vi "Module - Setting Page.vi"() -> ()   [LabVIEW 2020]
uses:
  Control/State - Setting.ctl
  Control/State - eFGV.ctl
  Control/Button Strip.ctl
  Control/Config File Selection.ctl
panel:
  out "error out":errorcluster
  in  "error in (no error)":errorcluster
  out "Site Name":string="SETTING"
  in  "MYSQL DATABASE":T1
  in  "MODBUS TCP IP":T2
  in  "setting_save_mysql":bool
  in  "setting_save":bool
  # "DB_CONNECTION :"
  # "DB_HOST :"
  # "DB_PORT  :"
  # "DB_DATABASE  :"
  # "DB_USERNAME  :"
  # "DB_PASSWORD  :"
  # "INTERVAL  :"
  # "SB-01"
  # "IP ADDRESS"
  # "PORT"
  # "SB-02"
  # "IP ADDRESS"
  # "PORT"
  # "SI-M"
  # "IP ADDRESS"
  # "PORT"
  # "SI-01"
  # "IP ADDRESS"
  # "PORT"
  # "DATA MANAGER"
  # "IP ADDRESS"
  # "PORT"
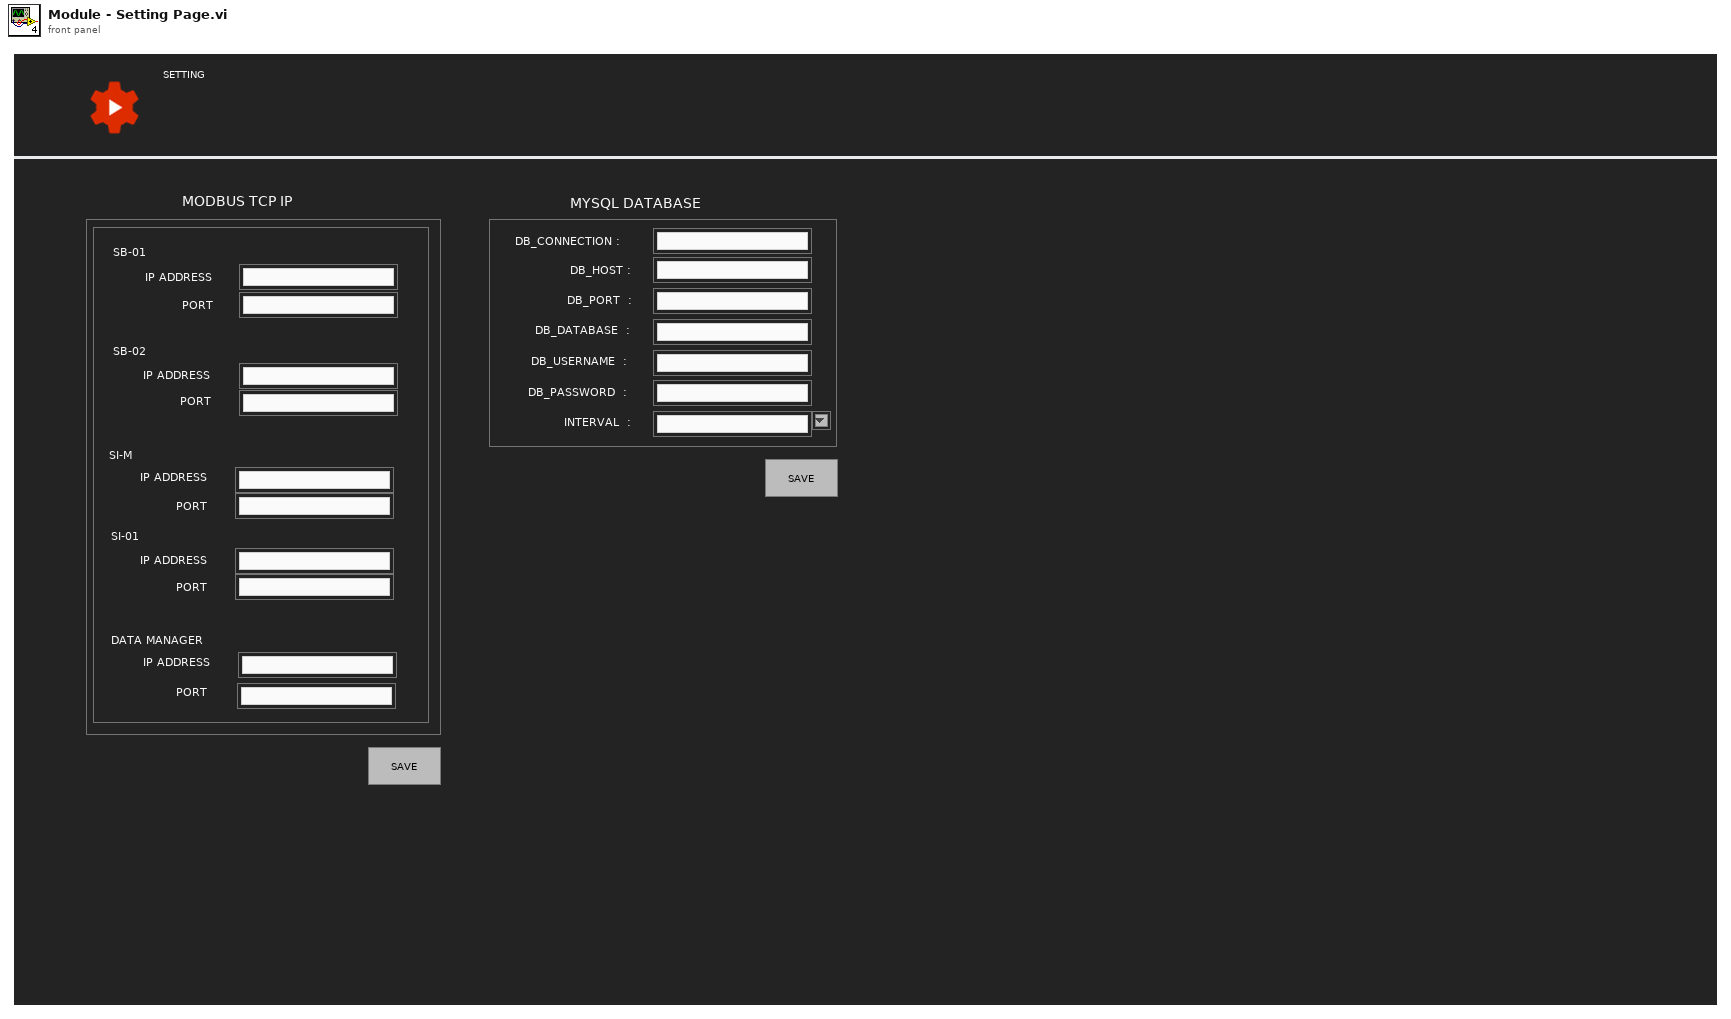
[diagram p1: front panel]
types:
  T1 = cluster{"db_connection":string, "db_host":string, "db_port":string, "db_database":string, "db_username":string, "db_pwd":string, "Interval":string}
  T2 = cluster{"DM-PORT":string, "DM-IPADDRESS":string, "SB-01-IPADDRESS":string, "SB-01-PORT":string, "SB-02-IPADDRESS":string, "SB-02-PORT":string, "SI-M-IPADDRESS":string, "SI-M-PORT":string, "SI-01-IPADDRESS":string, "SI-01-PORT":string}
  T3 = cluster{"Timeout":i32, "Modbus Config":string[][], "SQL Config":string[][]}
  T4 = typedef "State - Setting.ctl" = enum16{"Init module", "Register event", "Idle", "Read Config File", "Repopulate Indicator", "Save Modbus Settings", "Save SQL Settings", "Unregister event", "Close module"}
  T5 = typedef "Button Strip.ctl" = enum32{"Home", "Setting", "Alert", "Save", "Chart"}
  T6 = typedef "Config File Selection.ctl" = enum16{"Modbus", "SQL", "General"}
  T7 = typedef "State - eFGV.ctl" = enum16{"Init", "Read", "Write", "Close"}
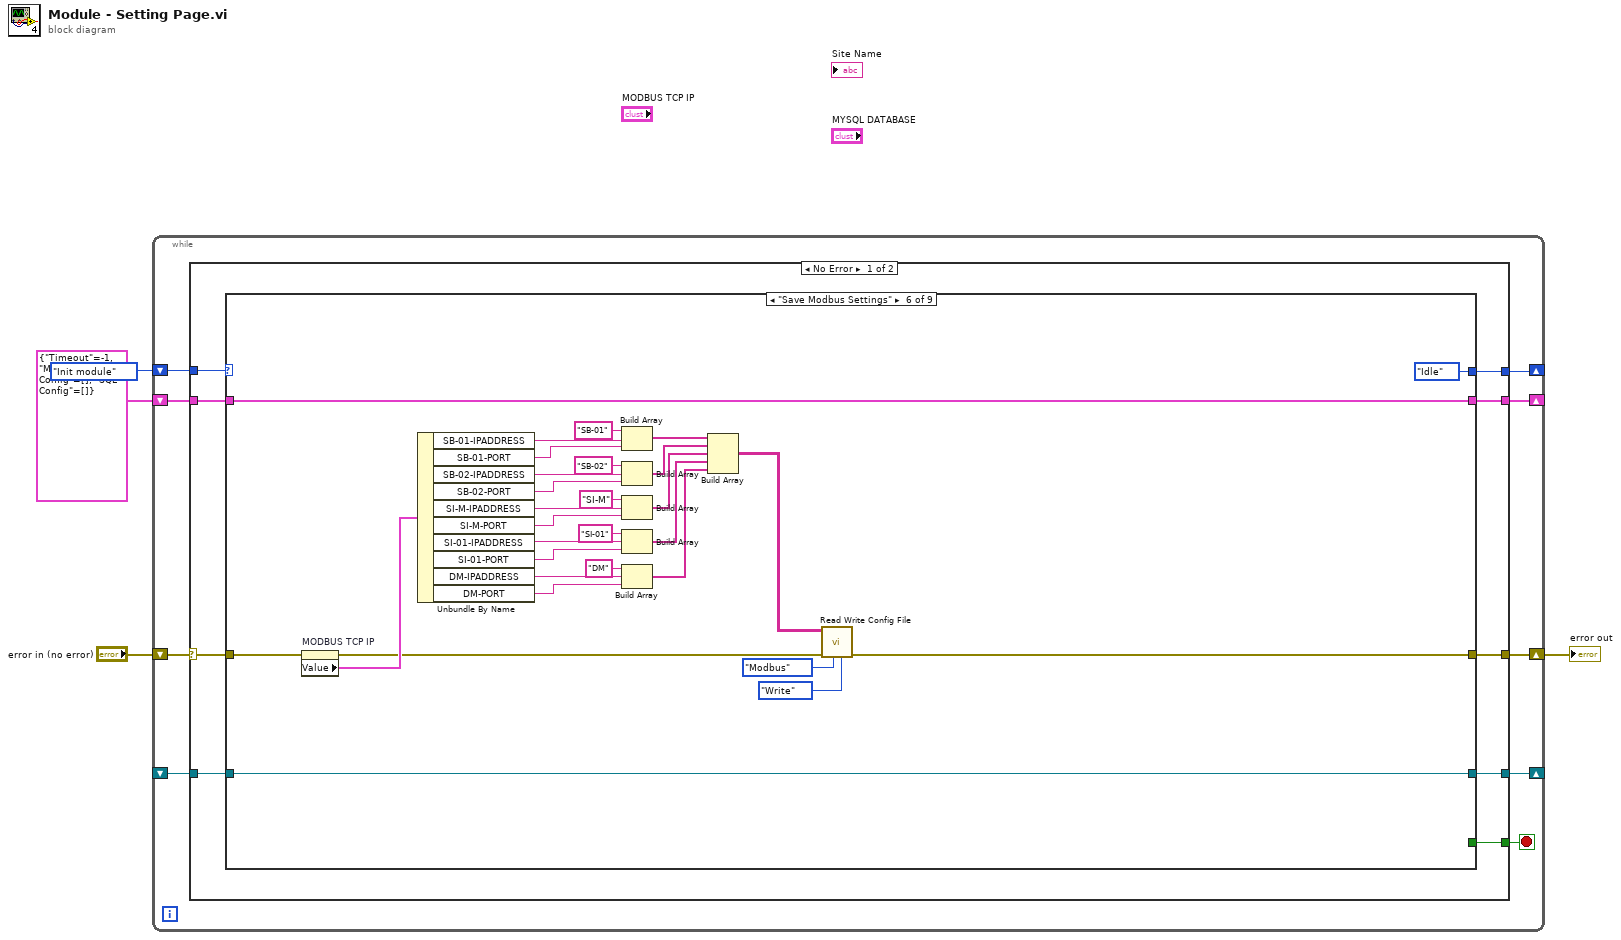
[diagram p0: block diagram]
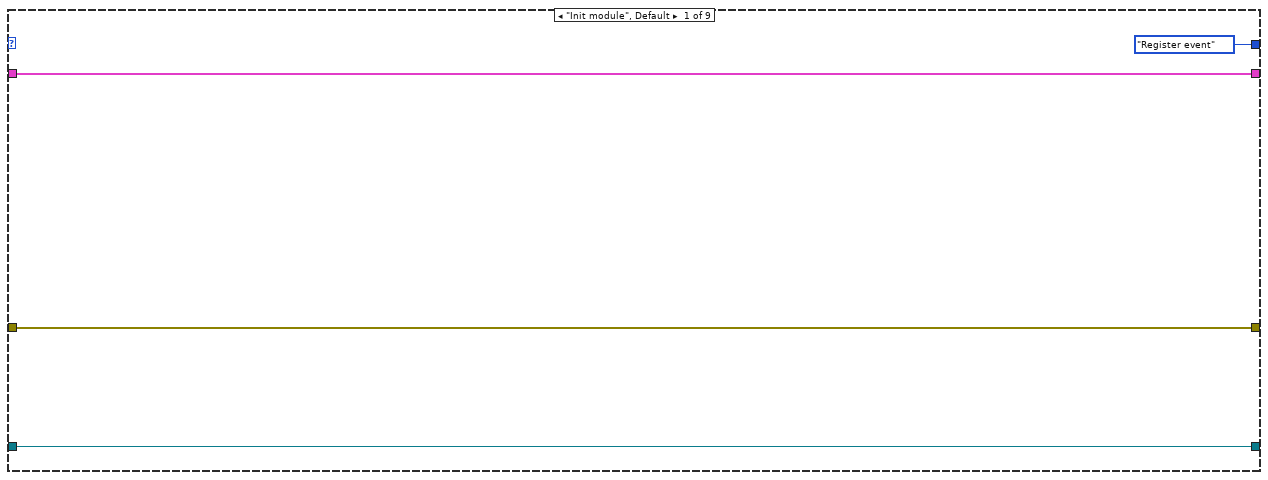
[diagram p2: hidden frame]
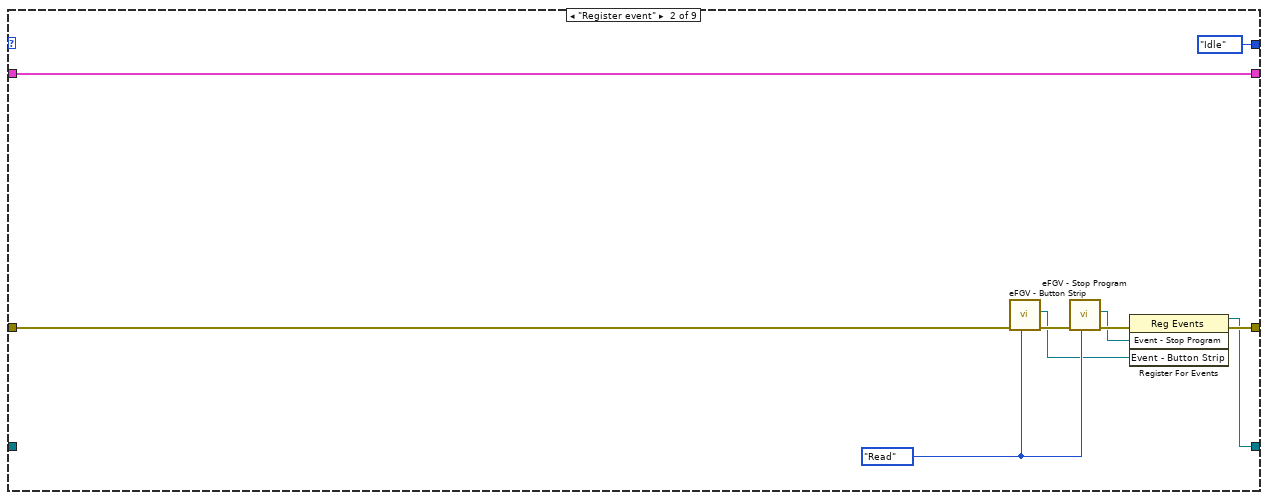
[diagram p3: hidden frame]
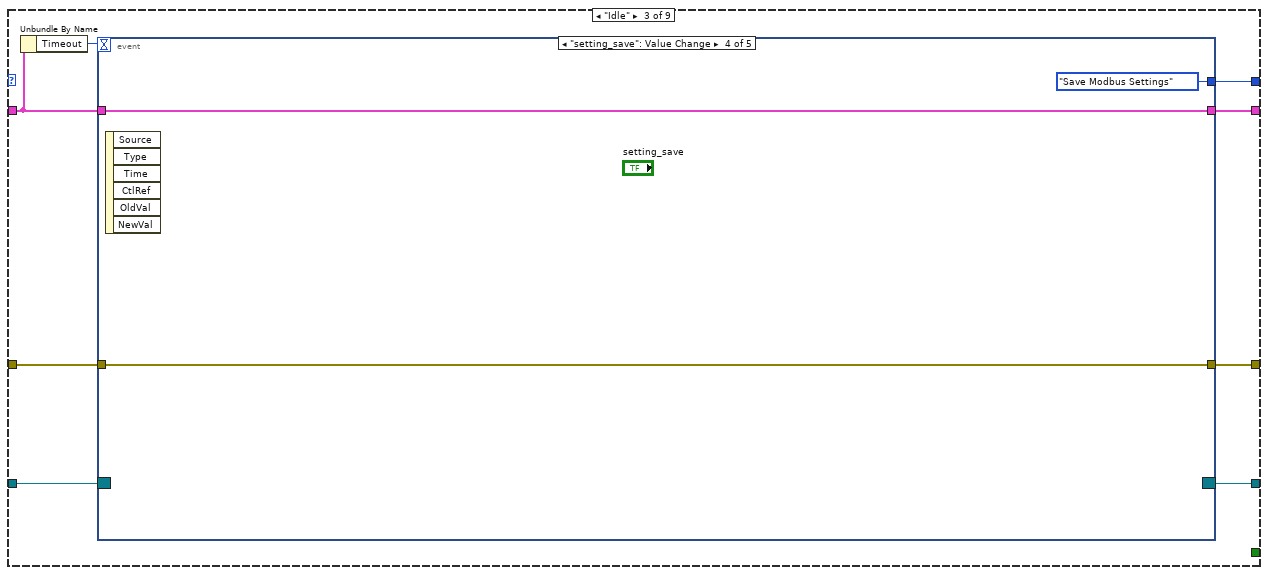
[diagram p4: hidden frame]
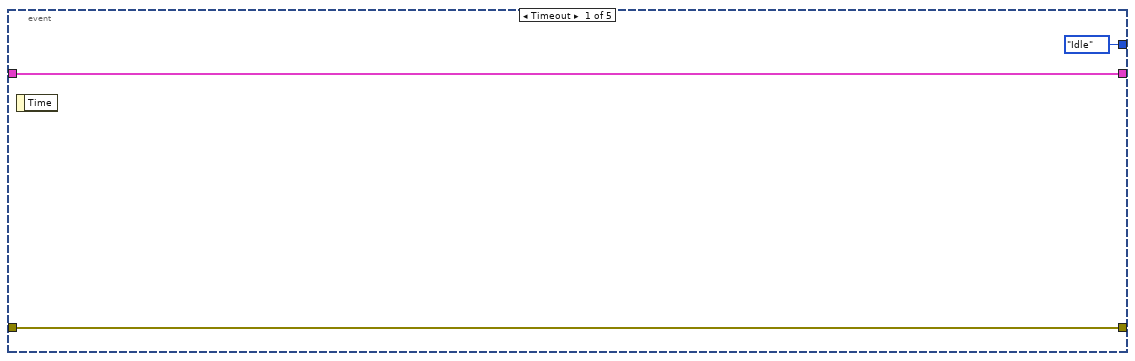
[diagram p5: hidden frame]
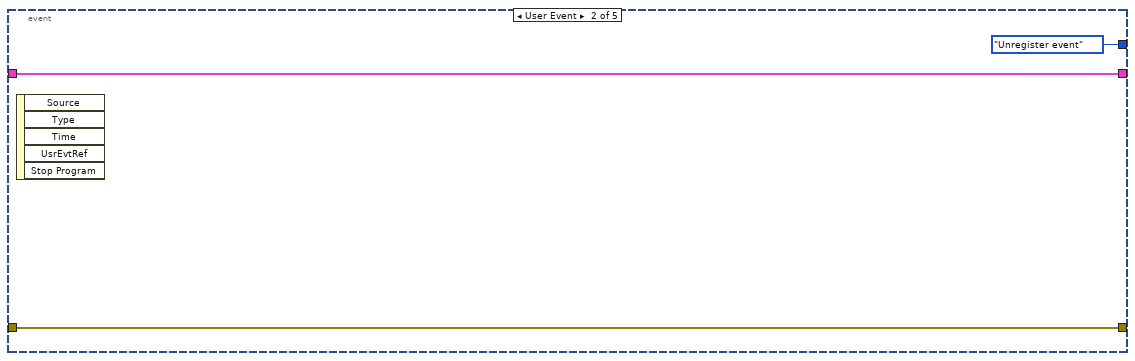
[diagram p6: hidden frame]
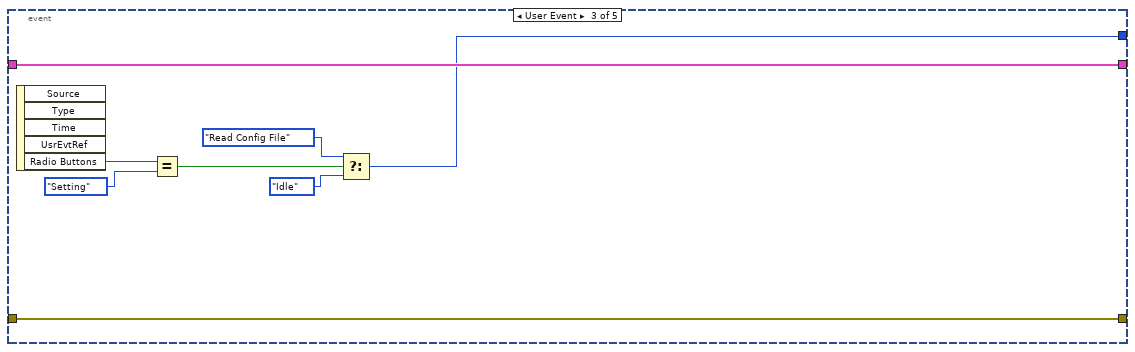
[diagram p7: hidden frame]
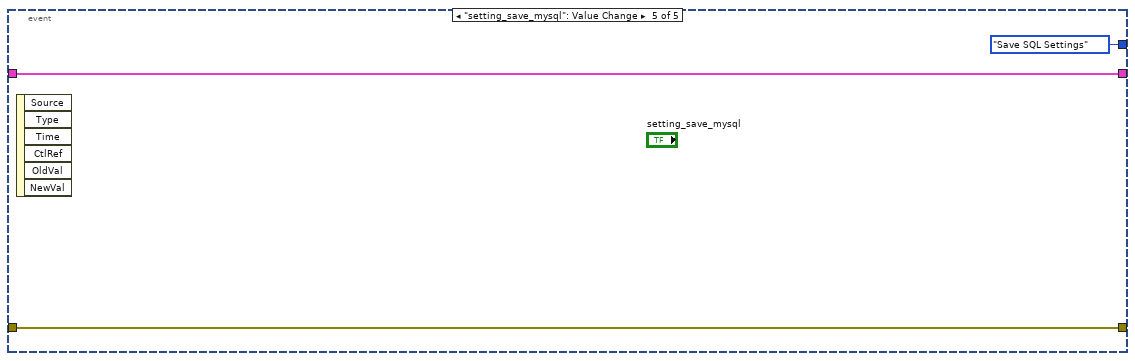
[diagram p8: hidden frame]
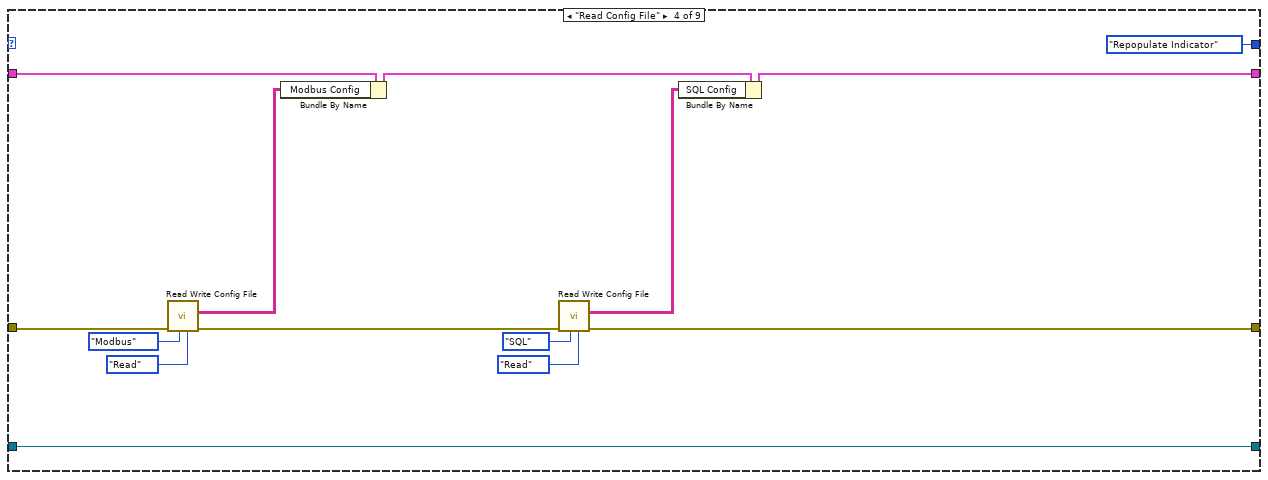
[diagram p9: hidden frame]
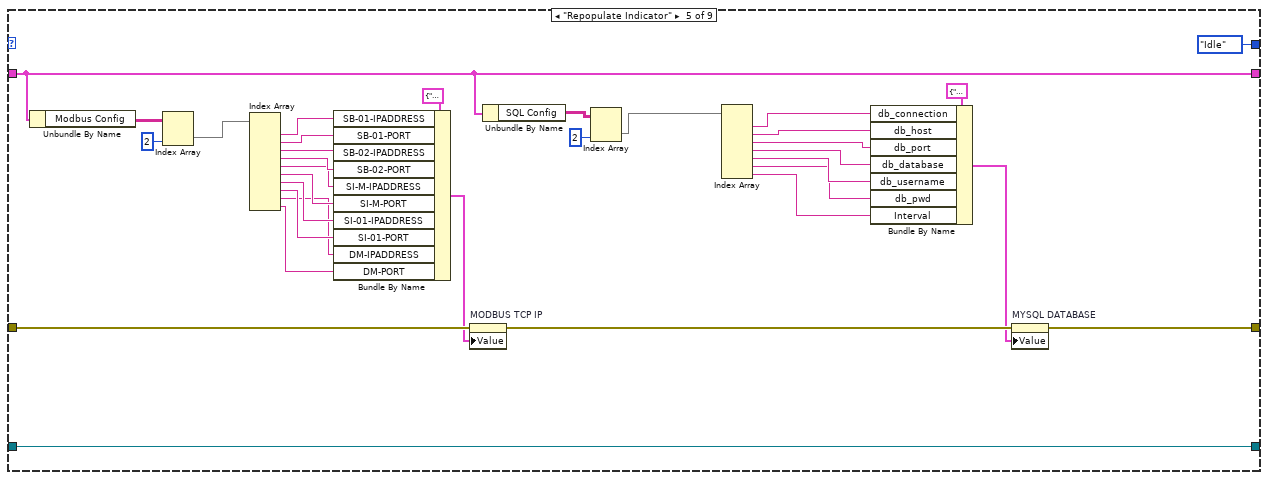
[diagram p10: hidden frame]
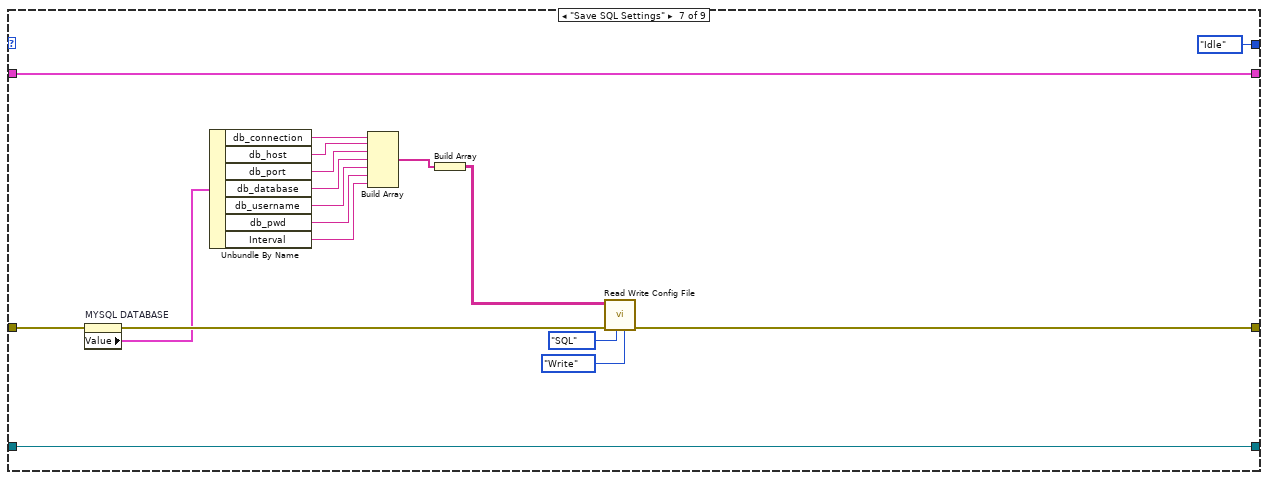
[diagram p11: hidden frame]
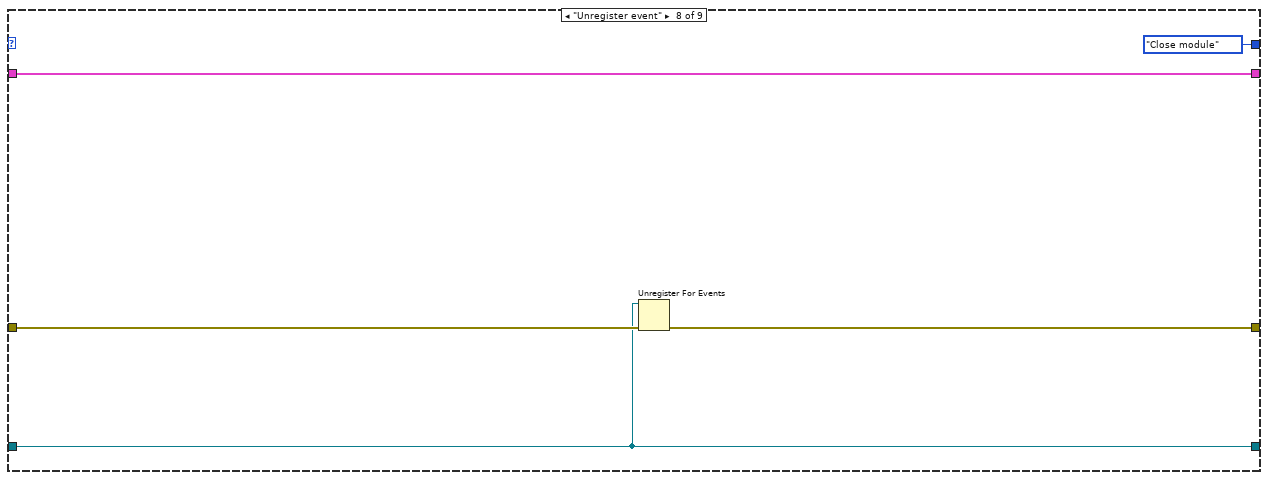
[diagram p12: hidden frame]
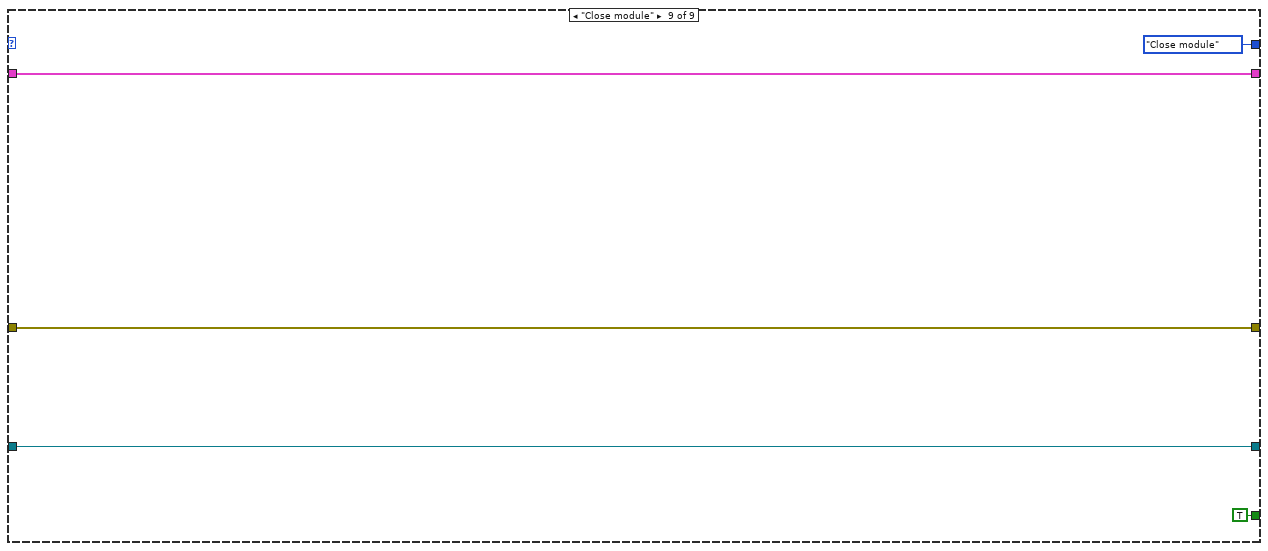
[diagram p13: hidden frame]
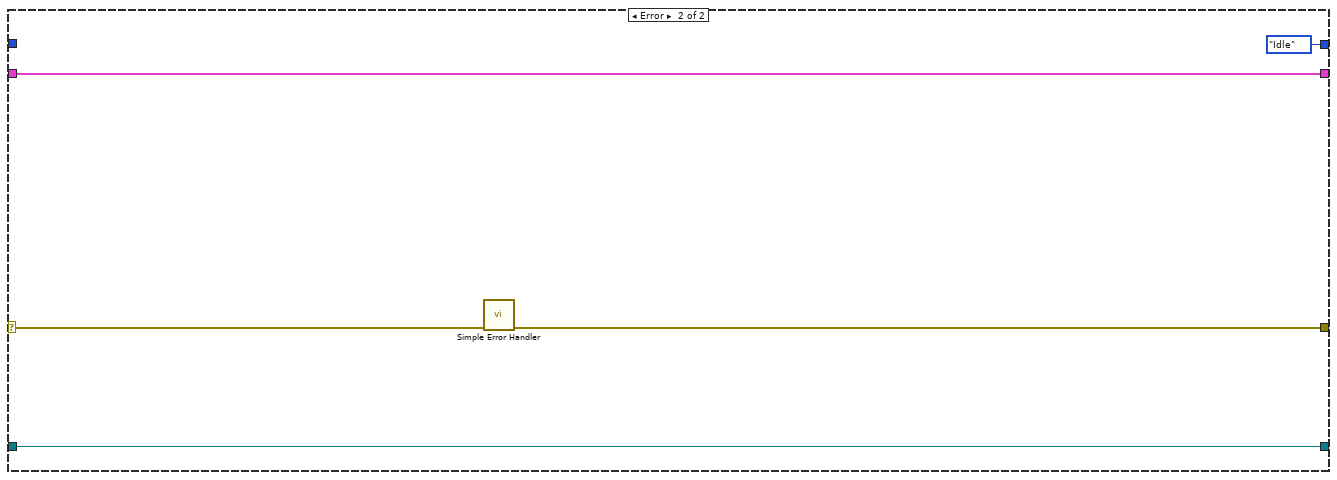
[diagram p14: hidden frame]
diagram:
  n1 = while {
    shift-right: [w11] -> w3
    shift-left: "error in (no error)" -> [w13]
    shift-right: [w5] -> _
    shift-left: State_-_Setting."Init module" -> [w12]
    shift-right: [w10] -> _
    shift-left: _ -> [w9]
    shift-right: [w7] -> _
    shift-left: T3 {"Timeout"=-1, "Modbus Config"=[], "SQL Config"=[]} -> [w8]
    stop <- w6 stop-if-true
    n2 = case shown="No Error" w13 {
      selector: w13 -> [w21 w174]
      tunnel: w12 -> [w22 _]
      tunnel: [w20 w173] -> w11
      tunnel: [w19 w172] -> w10
      tunnel: w9 -> [w18 w172]
      tunnel: w8 -> [w17 w171]
      tunnel: [w16 w171] -> w7
      tunnel: [w15 _] -> w6
      tunnel: [w14 State_-_Setting."Idle" ("f")] -> w5
      frame No Error {
        n3 = case shown="\"Save Modbus Settings\"" w22 {
          tunnel: w21 -> [w26 w30 w41 w76 w110 w139 w157 w163 w169]
          tunnel: [w26 w36 w38 w70 w93 w112 w152 w162 w169] -> w20
          tunnel: [w25 w35 w39 w78 w111 w141 w159 w161 w168] -> w19
          tunnel: w18 -> [w25 _ w40 w78 w111 w141 w159 w161 w168]
          tunnel: w17 -> [w24 w34 w43 w77 w92 w140 w158 w164 w167]
          tunnel: [w24 w34 w42 w67 w92 w140 w158 w164 w167] -> w16
          tunnel: [_ _ _ _ _ _ _ _ TRUE] -> w15
          tunnel: [State_-_Setting."Register event" State_-_Setting."Idle" w37 State_-_Setting."Repopulate Indicator" ("f") State_-_Setting."Idle" ("f") State_-_Setting."Idle" ("f") State_-_Setting."Idle" ("f") State_-_Setting."Close module" ("f") State_-_Setting."Close module" ("f")] -> w14
          frame "Init module", Default {
          }
          frame "Register event" {
            w29 = State_-_eFGV."Read" ("State - eFGV")
            n4 = call "eFGV - Button Strip.vi"("State - eFGV"=w29, "error in (no error)"=w30) -> ("error out"=w31:errorcluster, "Event - Button Strip"=w27:refnum<user-event>)  [unwired: 8 in]
            n5 = call "eFGV - Stop Program.vi"("State - eFGV"=w29, "error in (no error)"=w31) -> ("error out"=w32:errorcluster, "Event - Stop Program"=w28:refnum<user-event>)  [unwired: 8 in]
            n6 = register-events(error in=w32, w28, w27) -> (reference out=w35:refnum<event-registration>, error out=w36:errorcluster)  [unwired: 1 in]
          }
          frame "Idle" {
            n7 = Unbundle By Name(w43) -> ("Timeout"=w44:i32)
            n8 = event shown="[3] \"setting_save\": Value Change" {
              selector: w40 -> [_ _ _ _ _]
              dyn-events: [_ _ _ _ _] -> w39
              timeout: w44 -> [_ _ _ _ _]
              tunnel: w43 -> [w47 w49 w58 w61 w64]
              tunnel: [w47 w49 w58 w61 w64] -> w42
              tunnel: w41 -> [w46 w48 w52 w60 w63]
              tunnel: [w46 w48 w52 w60 w63] -> w38
              tunnel: [State_-_Setting."Idle" State_-_Setting."Unregister event" w51 State_-_Setting."Save Modbus Settings" ("f") State_-_Setting."Save SQL Settings" ("f")] -> w37
              event Timeout {
                n9 = event-data() -> ()  [unwired: 1 in, 1 out]
              }
              event User Event {
                n10 = event-data() -> ()  [unwired: 1 in, 5 out]
              }
              event User Event {
                n11 = event-data() -> ("Radio Buttons"=w57:T5)  [unwired: 1 in, 4 out]
                n12 = Equal?(x=w57, y=Button_Strip."Setting") -> (x = y?=w55:bool)
                n13 = Select(t=State_-_Setting."Read Config File", s=w55, f=State_-_Setting."Idle") -> (s? t:f=w51:T4)
              }
              event "setting_save": Value Change {
                n14 = event-data() -> ()  [unwired: 1 in, 6 out]
              }
              event "setting_save_mysql": Value Change {
                n15 = event-data() -> ()  [unwired: 1 in, 6 out]
              }
            }
          }
          frame "Read Config File" {
            n16 = call "Read Write Config File.vi"("Operation"=enum16{"Read", "Write"}."Read", "Config File"=Config_File_Selection."Modbus", "error in (no error)"=w76) -> ("error out"=w71:errorcluster, "Section-Key-Value Out"=w68:string[][])  [unwired: 7 in]
            n17 = Bundle By Name(cluster=w77, "Modbus Config"=w68) -> (w69:T3)
            n18 = call "Read Write Config File.vi"("Operation"=enum16{"Read", "Write"}."Read", "Config File"=Config_File_Selection."SQL", "error in (no error)"=w71) -> ("error out"=w70:errorcluster, "Section-Key-Value Out"=w66:string[][])  [unwired: 7 in]
            n19 = Bundle By Name(cluster=w69, "SQL Config"=w66) -> (w67:T3)
          }
          frame "Repopulate Indicator" {
            n20 = Unbundle By Name(w92) -> ("Modbus Config"=w84:string[][])
            n21 = Index Array(array=w84, index (col)=2 ("disabled index (col)")) -> (element=w82:string[])  [unwired: 1 in]
            n22 = Index Array(array=w82) -> (element #1=w106:string, element #2=w105:string, element #3=w104:string, element #4=w103:string, element #5=w102:string, element #6=w101:string, element #7=w100:string, element #8=w99:string, element #9=w98:string, element #10=w97:string)  [unwired: 10 in]
            n23 = Bundle By Name(cluster=T2 {"DM-PORT"="", "DM-IPADDRESS"="", "SB-01-IPADDRESS"="", "SB-01-PORT"="", "SB-02-IPADDRESS"="", "SB-02-PORT"="", "SI-M-IPADDRESS"="", "SI-M-PORT"="", "SI-01-IPADDRESS"="", "SI-01-PORT"=""} ("MODBUS TCP IP"), "SB-01-IPADDRESS"=w106, "SB-01-PORT"=w105, "SB-02-IPADDRESS"=w104, "SB-02-PORT"=w103, "SI-M-IPADDRESS"=w102, "SI-M-PORT"=w101, "SI-01-IPADDRESS"=w100, "SI-01-PORT"=w99, "DM-IPADDRESS"=w98, "DM-PORT"=w97) -> (w107:T2)
            n24 = property on="MODBUS TCP IP" class="Clust (strict)"(error in=w110, "Value"=w107) -> (error out=w109:errorcluster)  [unwired: 1 in, 1 out]
            n25 = Unbundle By Name(w92) -> ("SQL Config"=w81:string[][])
            n26 = Index Array(array=w81, index (col)=2 ("disabled index (col)")) -> (element=w79:string[])  [unwired: 1 in]
            n27 = Index Array(array=w79) -> (element #1=w91:string, element #2=w90:string, element #3=w89:string, element #4=w88:string, element #5=w87:string, element #6=w86:string, element #7=w85:string)  [unwired: 7 in]
            n28 = Bundle By Name(cluster=T1 {"db_connection"="", "db_host"="", "db_port"="", "db_database"="", "db_username"="", "db_pwd"="", "Interval"=""} ("MYSQL DATABASE"), "db_connection"=w91, "db_host"=w90, "db_port"=w89, "db_database"=w88, "db_username"=w87, "db_pwd"=w86, "Interval"=w85) -> (w95:T1)
            n29 = property on="MYSQL DATABASE" class="Clust (strict)"(error in=w109, "Value"=w95) -> (error out=w93:errorcluster)  [unwired: 1 in, 1 out]
          }
          frame "Save Modbus Settings" {
            n30 = property on="MODBUS TCP IP" class="Clust (strict)"(error in=w139) -> (error out=w114:errorcluster, "Value"=w138:T2)  [unwired: 1 in, 1 out]
            n31 = Unbundle By Name(w138) -> ("SB-01-IPADDRESS"=w137:string, "SB-01-PORT"=w136:string, "SB-02-IPADDRESS"=w135:string, "SB-02-PORT"=w134:string, "SI-M-IPADDRESS"=w133:string, "SI-M-PORT"=w132:string, "SI-01-IPADDRESS"=w131:string, "SI-01-PORT"=w130:string, "DM-IPADDRESS"=w129:string, "DM-PORT"=w128:string)
            n32 = Build Array("SB-01" ("element"), w137, w136) -> (w122:string[])
            n33 = Build Array("SB-02" ("element"), w135, w134) -> (w121:string[])
            n34 = Build Array("SI-M" ("element"), w133, w132) -> (w120:string[])
            n35 = Build Array("SI-01" ("element"), w131, w130) -> (w119:string[])
            n36 = Build Array("DM" ("element"), w129, w128) -> (w118:string[])
            n37 = Build Array(w122, w121, w120, w119, w118) -> (w113:string[][])
            n38 = call "Read Write Config File.vi"("Operation"=enum16{"Read", "Write"}."Write", "Config File"=Config_File_Selection."Modbus", "error in (no error)"=w114, "Section-Key-Value In"=w113) -> ("error out"=w112:errorcluster)  [unwired: 6 in, 1 out]
          }
          frame "Save SQL Settings" {
            n39 = property on="MYSQL DATABASE" class="Clust (strict)"(error in=w157) -> (error out=w153:errorcluster, "Value"=w151:T1)  [unwired: 1 in, 1 out]
            n40 = Unbundle By Name(w151) -> ("db_connection"=w150:string, "db_host"=w149:string, "db_port"=w148:string, "db_database"=w147:string, "db_username"=w146:string, "db_pwd"=w145:string, "Interval"=w144:string)
            n41 = Build Array(w150, w149, w148, w147, w146, w145, w144) -> (w143:string[])
            n42 = Build Array(w143) -> (w142:string[][])
            n43 = call "Read Write Config File.vi"("Operation"=enum16{"Read", "Write"}."Write", "Config File"=Config_File_Selection."SQL", "error in (no error)"=w153, "Section-Key-Value In"=w142) -> ("error out"=w152:errorcluster)  [unwired: 6 in, 1 out]
          }
          frame "Unregister event" {
            n44 = Unregister For Events(event registration refnum=w161, error in=w163) -> (error out=w162:errorcluster)
          }
          frame "Close module" {
          }
        }
      }
      frame Error {
        n45 = call <vilib>:"Simple Error Handler.vi"("error in (no error)"=w174) -> ("error out"=w173:errorcluster)  [unwired: 4 in, 4 out]
      }
    }
  }
  "error out" <- w3
